vi "upload_session_append.vi"(6 "timeout_ms":i32=10000, 8 "error in (no error)":errorcluster, 9 "offset":i64, 10 "data":string, 11 "session_id":string) -> (0 "error out":errorcluster)   [LabVIEW 2015, in "lv-dropbox.lvlib" / "v2.lvlib"]
uses:
  v2.lvlib
  private/_controls/content_type.ctl
  <vilib>/httpClient/POSTBuffer.vi
  <vilib>/httpClient/LabVIEWHTTPClient.lvlib
  lv-dropbox.lvlib
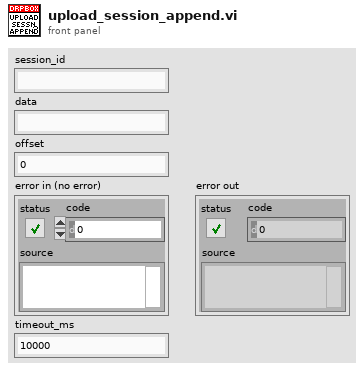
[diagram p1: front panel]
types:
  T1 = typedef "lv-dropbox.lvlib/content_type.ctl" = enum16{"<content_type>", "json", "application/octet-stream"}
  T2 = typedef "LabVIEWHTTPClient.lvlib/ClientHandle.ctl" = refnum<k1>
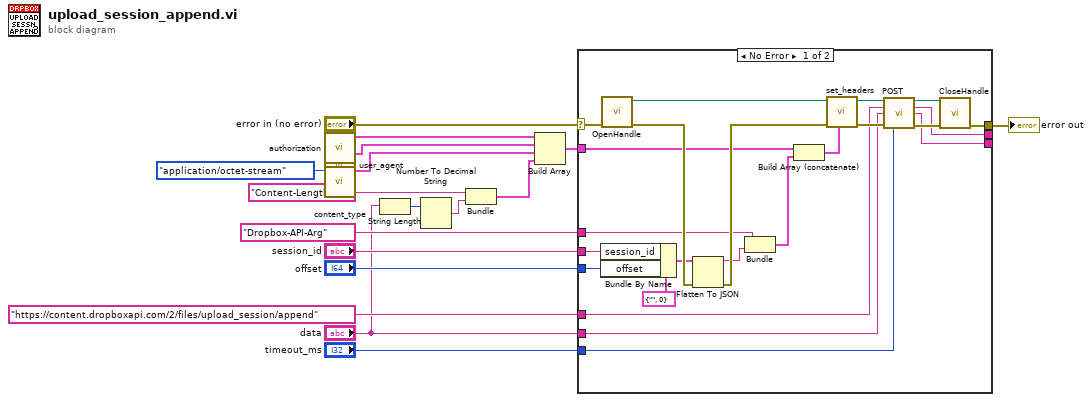
[diagram p0: block diagram]
diagram:
  n1 = call "authorization.vi"() -> ("header"=w13:cluster{"header":string, "value":string})  [unwired: 11 in]
  n2 = call "user_agent.vi"() -> ("header"=w16:cluster{"header":string, "value":string})  [unwired: 11 in]
  n3 = call "content_type.vi"("content_type"=content_type."application/octet-stream") -> ("header"=w17:cluster{"header":string, "value":string})  [unwired: 10 in]
  n4 = String Length(string="data") -> (length=w3:i32)
  n5 = Number To Decimal String(number=w3) -> (decimal integer string=w5:string)  [unwired: 1 in]
  n6 = Bundle("header"="Content-Length", w5) -> (w6:cluster{"header":string, string})  [unwired: 1 in]
  n7 = Build Array(w13, w16, w17, w6) -> (w12:cluster{"header":string, "value":string}[])
  n8 = case shown="No Error" "error in (no error)" {
    selector: "error in (no error)" -> [w33 w41]
    tunnel: w12 -> [w32 _]
    tunnel: "https://content.dropboxapi.com/2/files/upload_session/append" ("url") -> [w31 _]
    tunnel: [w38 w41] -> w1
    tunnel: "session_id" -> [w29 _]
    tunnel: "offset" -> [w28 _]
    tunnel: "Dropbox-API-Arg" ("header") -> [w26 _]
    tunnel: "timeout_ms" -> [w22 _]
    tunnel: "data" -> [w21 _]
    tunnel: [w19 _] -> _
    tunnel: [w18 _] -> _
    frame No Error {
      n9 = Bundle By Name(cluster=cluster{"session_id":string, "offset":i64} {"session_id"="", "offset"=0}, "session_id"=w29, "offset"=w28) -> (w27:cluster{"session_id":string, "offset":i64})
      n10 = call <vilib>:"OpenHandle.vi"("error in (no error)"=w33) -> ("client handle out"=w36:T2, "error out"=w40:errorcluster)  [unwired: 13 in]
      n11 = Flatten To JSON(anything=w27, error in (no error)=w40) -> (JSON string=w25:string, 11:w39:errorcluster)  [unwired: 1 in]
      n12 = Bundle("header"=w26, "JSON string"=w25) -> (w24:cluster{"header":string, "JSON string":string})  [unwired: 1 in]
      n13 = Build Array (concatenate)(w32, w24) -> (w30:cluster{"header":string, "JSON string":string}[])
      n14 = call "set_headers.vi"("header_value []"=w30, "error in (no error)"=w39, "client_handle in"=w36) -> ("error out"=w34:errorcluster, "client_handle out"=w35:T2)  [unwired: 7 in]
      n15 = call-poly <vilib>:"POST.vi"("client handle"=w35, "url"=w31, "buffer"=w21, "error in (no error)"=w34, "timeout (10000)"=w22) -> ("client handle out"=w37:T2, "headers"=w19:string, "body"=w18:string, "error out"=w20:errorcluster)  [unwired: 7 in]
      n16 = call <vilib>:"CloseHandle.vi"("client handle"=w37, "error in (no error)"=w20) -> ("error out"=w38:errorcluster)  [unwired: 13 in]
    }
    frame Error {
    }
  }
  "error out" <- w1
